vi "Bounds to Corner Positions.vi"(11 "bounds":T2) -> (2 "bottom right":T1, 3 "top left":T1)   [LabVIEW 2010, in "NI_SE_Front Panel Layout.lvlib"]
uses:
  NI_SE_Front Panel Layout.lvlib
  <vilib>/Utility/miscctls.llb/LVRectTypeDef.ctl
  <vilib>/Utility/miscctls.llb/LVPointTypeDef.ctl
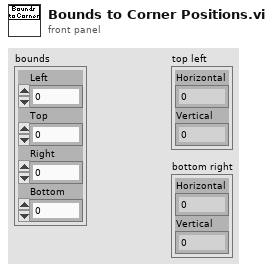
[diagram p1: front panel]
types:
  T1 = typedef "LVPointTypeDef.ctl" = cluster{"Horizontal":i16, "Vertical":i16}
  T2 = typedef "LVRectTypeDef.ctl" = cluster{"Left":i16, "Top":i16, "Right":i16, "Bottom":i16}
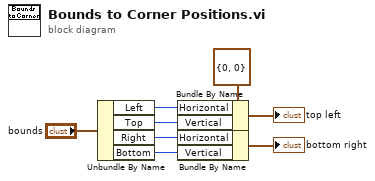
[diagram p0: block diagram]
diagram:
  w4 = T1 {"Horizontal"=0, "Vertical"=0} ("Point")
  n1 = Unbundle By Name("bounds") -> ("Left"=w6:i16, "Top"=w5:i16, "Right"=w3:i16, "Bottom"=w2:i16)
  n2 = Bundle By Name(cluster=w4, "Horizontal"=w6, "Vertical"=w5) -> (→"top left":T1)
  n3 = Bundle By Name(cluster=w4, "Horizontal"=w3, "Vertical"=w2) -> (→"bottom right":T1)
